vi "FPGA Write FIFO By Name - U8.vi"(6 "Timeout (ms)":u32, 8 "error in (no error)":errorcluster, 9 "Data":u8[](array[numeric]), 10 "FIFO":string, 11 "FPGA Session In":refnum<class "FPGA Interface Base.lvclass">) -> (0 "error out":errorcluster, 1 "Empty Elements Remaining":u32, 3 "FPGA Session Out":refnum<class "FPGA Interface Base.lvclass">)   [LabVIEW 2010, in "FPGA Interface Base.lvclass"]
doc: "Writes to a FIFO of unsigned 8-bit integers."
uses:
  <userlib>/_FPGA Interface Advanced Tools/FPGA Interface Base/FPGA Interface Base.lvclass
  <vilib>/rvi/DataTransferAndStorage/Container/Common/niFpgaDataTypeControl.ctl
  <userlib>/_FPGA Interface Advanced Tools/FPGA Interface Base/FPGA Interface Base.lvclass/FPGA Interface Base.ctl
  <vilib>/Utility/error.llb/Error Cluster From Error Code.vi
  <userlib>/_FPGA Interface Advanced Tools/FPGA Interface Base/Accessors/FPGA Read Session.vi
  <userlib>/_FPGA Interface Advanced Tools/FPGA Interface Wrapper/FPGA Interface Wrapper.lvlib
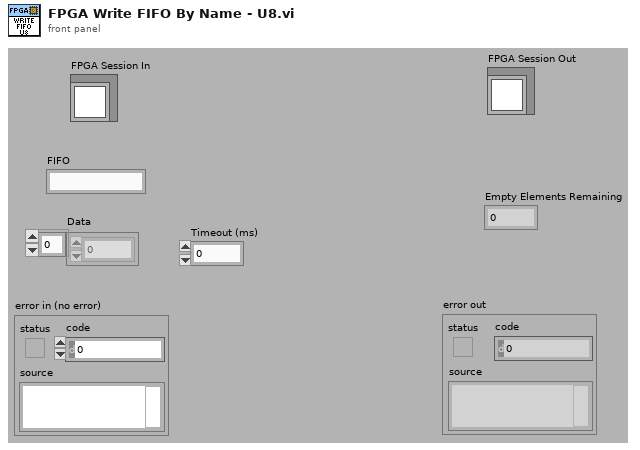
[diagram p1: front panel]
types:
  T1 = typedef "niFpgaDataTypeControl.ctl" = enum32{"Boolean", "I8", "I16", "I32", "I64", "U8", "U16", "U32", "U64", "FXP", "CustomControl"}
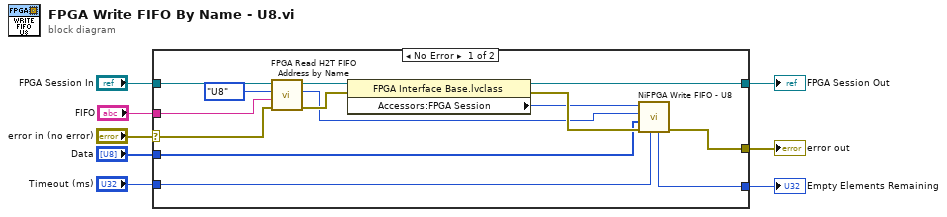
[diagram p0: block diagram]
diagram:
  n1 = case shown="No Error" "error in (no error)" {
    selector: "error in (no error)" -> [w15 w24]
    tunnel: [w19 w24] -> w7
    tunnel: [w20 w23] -> w8
    tunnel: "FPGA Session In" -> [w11 w23]
    tunnel: "FIFO" -> [w13 _]
    tunnel: [w18 _] -> w6
    tunnel: "Data" -> [w17 _]
    tunnel: "Timeout (ms)" -> [w16 _]
    frame No Error {
      n2 = call <userlib>:"FPGA Read H2T FIFO Address by Name.vi"("error in (no error)"=w15, "Name"=w13, "Data Type"=niFpgaDataTypeControl."U8", "FPGA Interface Base in"=w11) -> ("error out"=w14:errorcluster, "Address"=w9:u32, "FPGA Interface Base out"=w10:refnum<class "FPGA Interface Base.lvclass">)  [unwired: 4 in, 1 out]
      n3 = property class="FPGA Interface Base.lvclass"(reference=w10, error in=w14) -> (reference out=w20:refnum<class "FPGA Interface Base.lvclass">, error out=w22:errorcluster, "Accessors:FPGA Session"=w21:u32)
      n4 = call <userlib>:"NiFPGA Write FIFO - U8.vi"("Timeout"=w16, "error in (no error)"=w22, "Data"=w17, "FIFO"=w9, "Session"=w21) -> ("error out"=w19:errorcluster, "Empty Elements Remaining"=w18:u32)  [unwired: 4 in, 1 out]
    }
    frame Error {
    }
  }
  "error out" <- w7
  "FPGA Session Out" <- w8
  "Empty Elements Remaining" <- w6
